vi "IP Units tester V1.vi"() -> ()   [LabVIEW 2015]
uses:
  IP Dev Area/IP results.ctl
  <vilib>/FPGAPlugInAG/Dynamic/niLvFpga_Reset_Dynamic.vi
  <vilib>/FPGAPlugInAG/Dynamic/niLvFpga_Abort_Dynamic.vi
  <vilib>/FPGAPlugInAG/Dynamic/niLvFpga_Run_Dynamic.vi
  <vilib>/Utility/error.llb/Error Cluster From Error Code.vi
  <vilib>/rvi/errors/niLvFpgaAdjustHostInterfaceError.vi
  <vilib>/rvi/interface/common/niFpgaWaitOnOcc.vi
  <vilib>/rvi/interface/nirviMethod/nirviMethod.xnode
  <vilib>/rvi/interface/nirviReadWriteControl/nirviReadWriteControl.xnode
  <vilib>/vision/NI_Vision_Development_Module.lvlib
  <vilib>/rvi/interface/nirviOpenFPGA/nirviOpenFPGA.xnode
  <vilib>/visionFPGA/NI_VDM_FPGA_Basics.lvlib
  <vilib>/visionFPGA/Basics/Configure Image Transfer from Target/IMAQ FPGA Configure Image Transfer from Target U8.vi
  <vilib>/visionFPGA/Basics/Configure Image Transfer to Target/IMAQ FPGA Configure Image Transfer to Target U8.vi
  <vilib>/visionFPGA/Basics/Image Transfer from Target/IMAQ FPGA Image Transfer from Target U8.vi
  <vilib>/rvi/errors/niLvFpgaMergeErrorWithErrorCode.vi
  <vilib>/FPGAPlugInAG/Dynamic/niLvFpga_ConfigureFifo_Dynamic.vi
  <vilib>/FPGAPlugInAG/Dynamic/niLvFpga_StartFifo_Dynamic.vi
  <vilib>/rvi/interface/Simulation/niFpgaSimulationCallBeginRW.vi
  <vilib>/FPGAPlugInAG/Dynamic/niLvFpga_StopFifo_Dynamic.vi
  <vilib>/FPGAPlugInAG/Dynamic/niLvFpga_ReadFifo_Dynamic.vi
  NiFpgaLv.dll
  <vilib>/FPGAPlugInAG/Dynamic/niLvFpga_WriteFifo_Dynamic.vi
  IP Dev Area/FPGA IP Chain V1.vi
  <vilib>/rvi/interface/RandomDataEmulation/nirviRandomDataOpen.vi
  <vilib>/rvi/interface/common/niFpgaCacheSessionInfoDynamic.vi
panel:
  out "SuspPixelsX":u32[](array[numeric])
  out "IP Results":T1
  out "Y Points":i16[](array[numeric])
  out "X Points":i16[](array[numeric])
  out "SuspPixelsIndex":u32[](array[numeric])=[25, 34, 37, 42, 47, 52, 57, 63, 66, 75]
  out "Intensity Graph":u8[][](graph)
  out "ApCounter":u32
  out "Yaccum":u32
  out "Xaccum":u32
  out "counter":u32
  out "error out 7":errorcluster
  out "lo(x)":u16[](array[numeric])
  out "hi(x)":u16[](array[numeric])
  out "error out 6":errorcluster
  out "Results":u32[](array[numeric])
  out "transposed array 2":u8[][](array[numeric])
  out "error out 5":errorcluster
  out "transposed array":u8[][](graph)
  out "error out 4":errorcluster
  out "error out 3":errorcluster
  out "error out 2":errorcluster
  out "error out":errorcluster
  out "Image Out":T2(plugin-control)
  in  "Image Dir Path":path=path "D:/Dropbox (Testview)/Shared Projects/BELKIN Software/Eagle Software/Eagle Code/EyePictures/DebugPics" caption="Image Path"
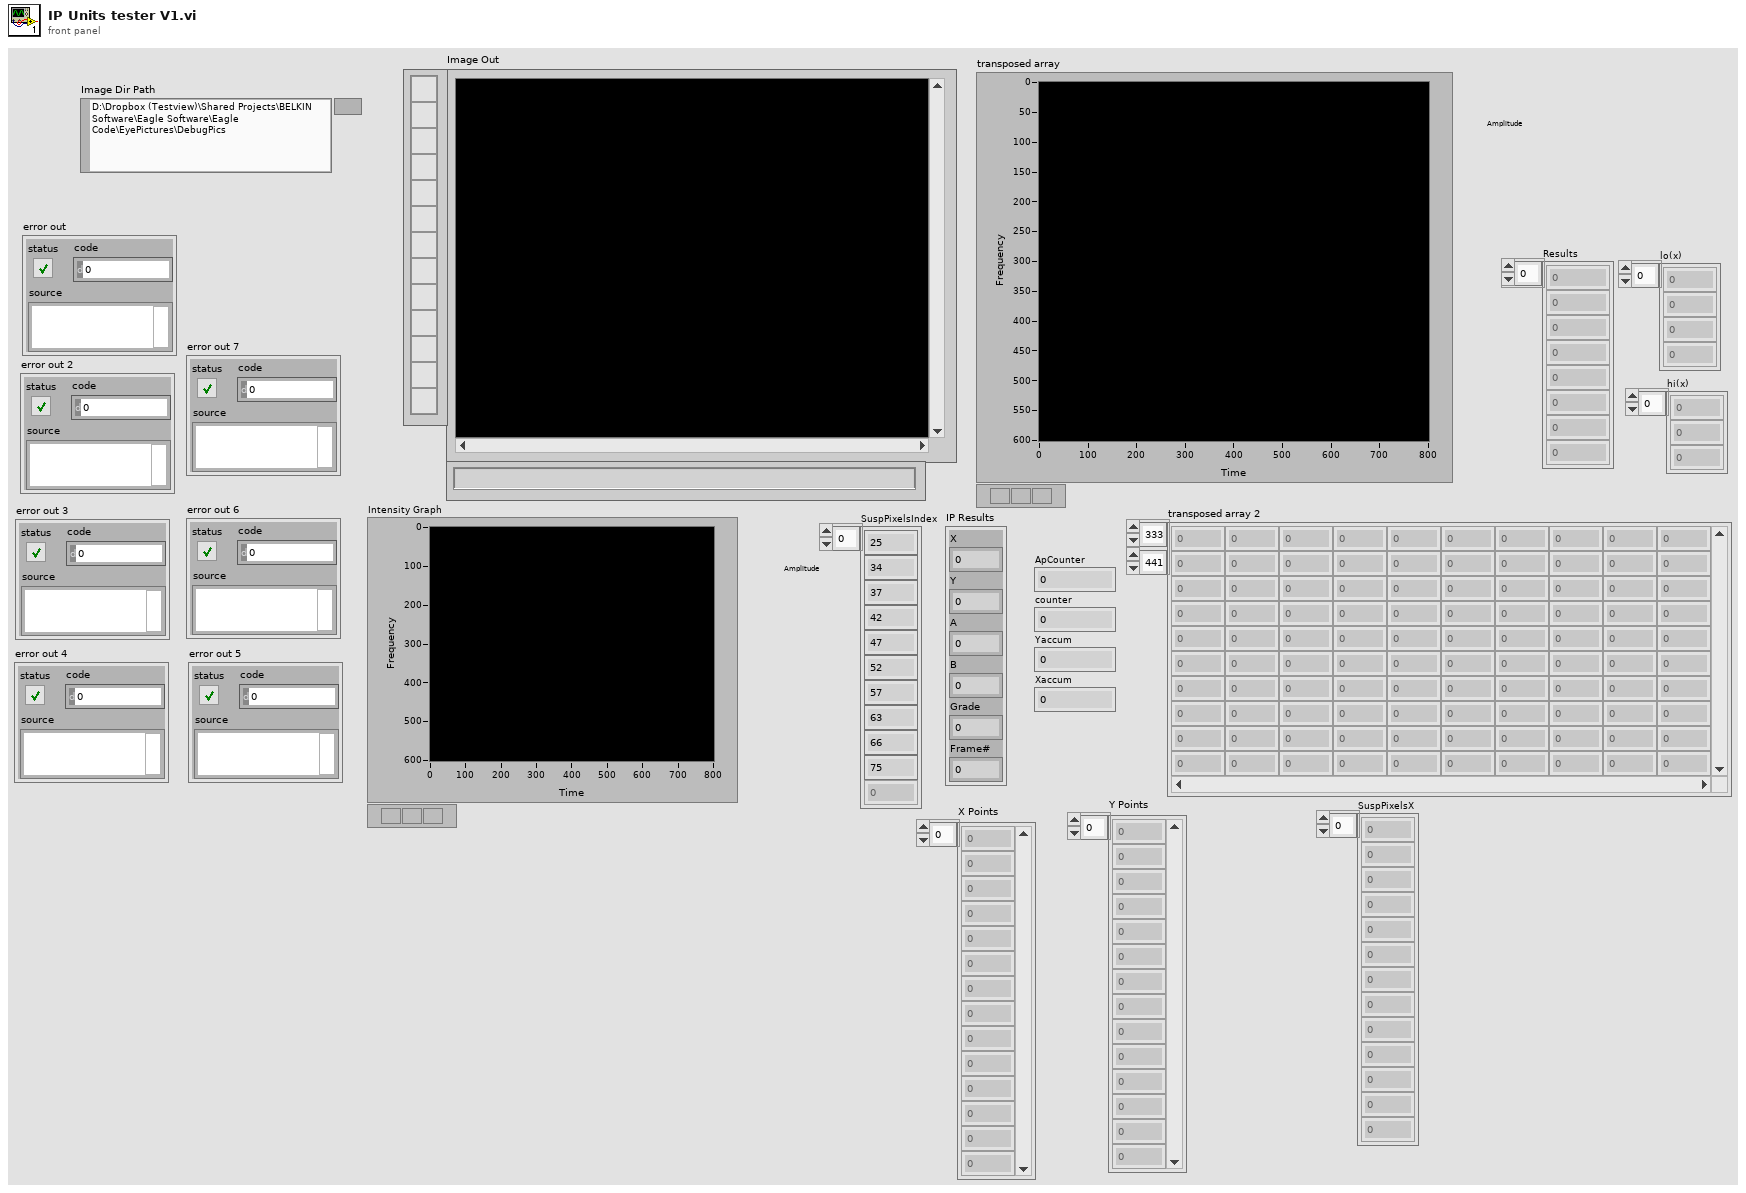
[diagram p1: front panel]
types:
  T1 = typedef "IP results.ctl" = cluster{"X":u16, "Y":u16, "A":dbl, "B":dbl, "Grade":u16, "Frame#":u16}
  T2 = typedef "IMAQ Image.ctl" = refnum<image>
  T3 = typedef "Image Type" = u32
  T4 = cluster{"DMA FIFO Name":string, "Image Size Control Name":string}
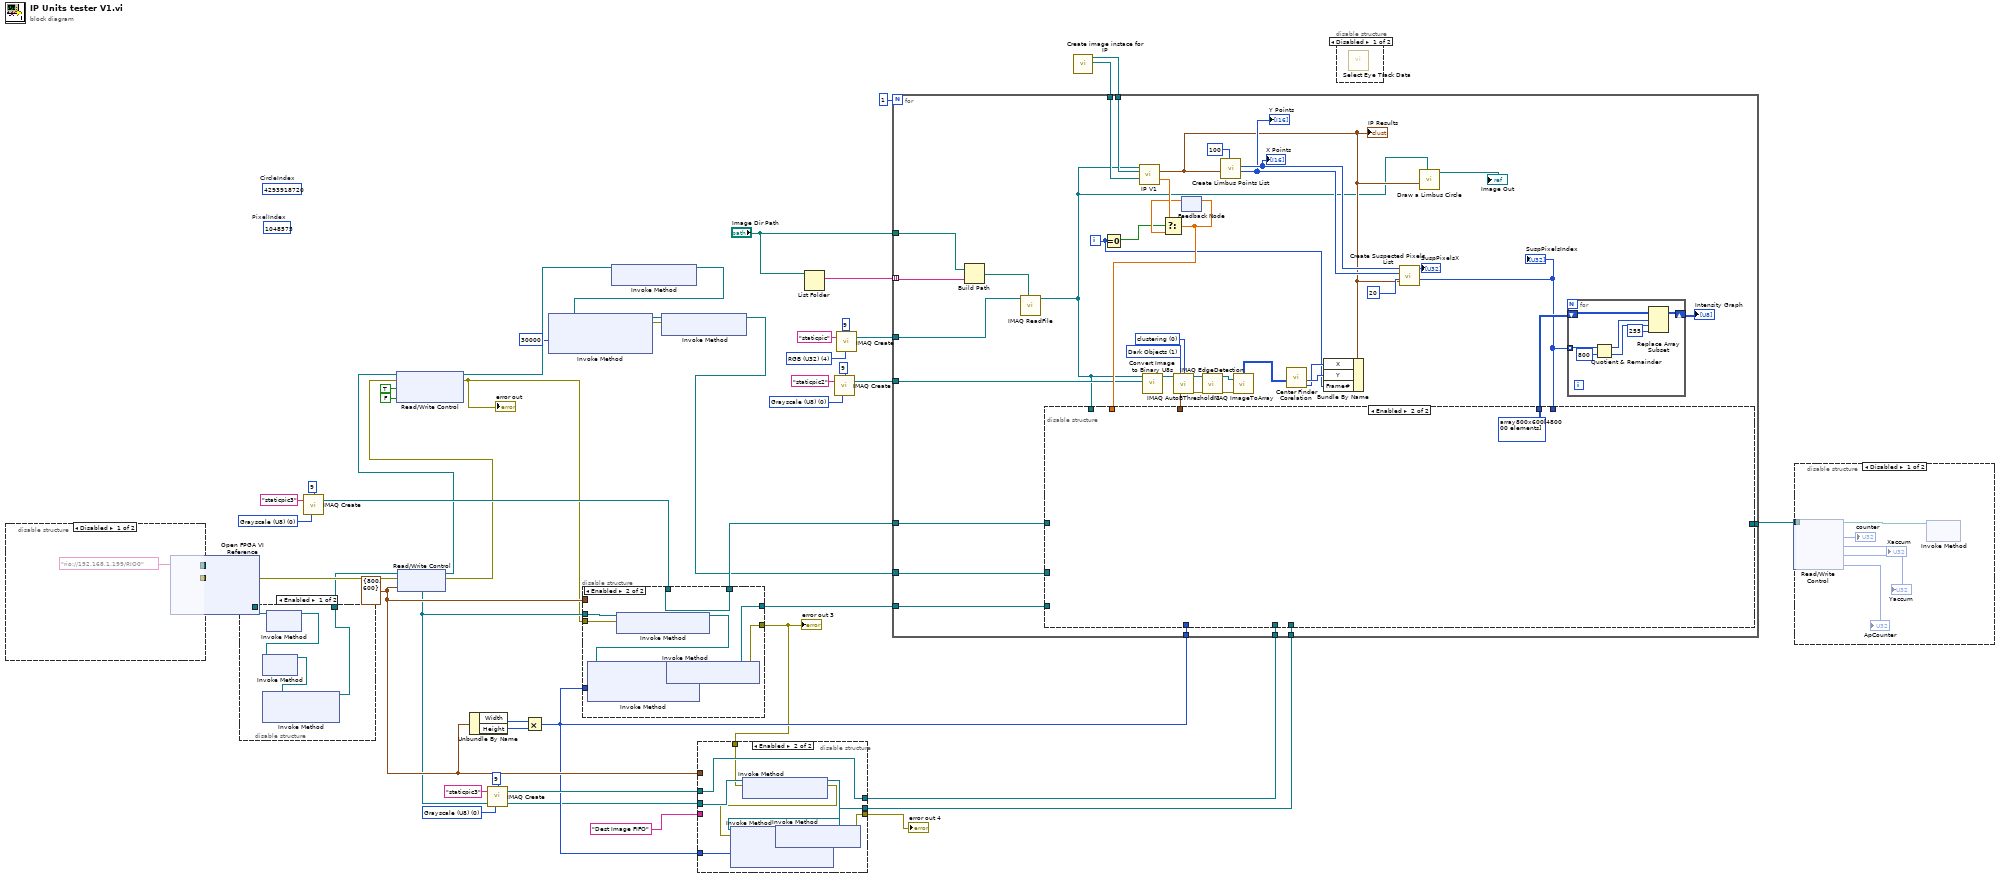
[diagram p0: block diagram]
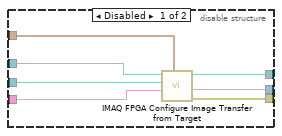
[diagram p6: hidden frame]
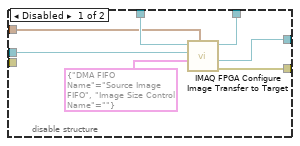
[diagram p7: hidden frame]
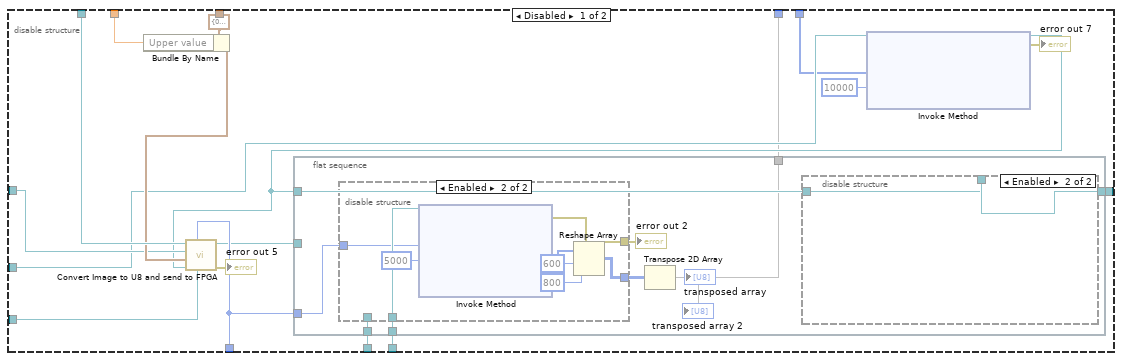
[diagram p8: hidden frame]
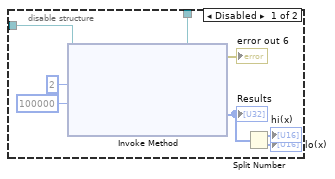
[diagram p9: hidden frame]
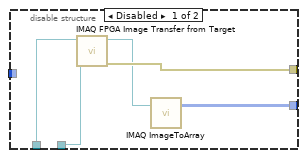
[diagram p10: hidden frame]
diagram:
  (unwired) u32 4293918720  # CircleIndex
  (unwired) u32 1048575  # PixelIndex
  w26 = T3 0 items=["Grayscale (U8)", "Grayscale (I16)", "Grayscale (SGL)", "Complex (CSG)", "RGB (U32)", "HSL (U32)", "RGB (U64)", "Grayscale (U16)"] ("Image Type")
  w19 = cluster{"Width":u32, "Height":u32} {"Width"=800, "Height"=600} ("Image Size")
  w33 = T3 0 items=["Grayscale (U8)", "Grayscale (I16)", "Grayscale (SGL)", "Complex (CSG)", "RGB (U32)", "HSL (U32)", "RGB (U64)", "Grayscale (U16)"] ("Image Type")
  w37 = T3 0 items=["Grayscale (U8)", "Grayscale (I16)", "Grayscale (SGL)", "Complex (CSG)", "RGB (U32)", "HSL (U32)", "RGB (U64)", "Grayscale (U16)"] ("Image Type")
  w44 = T3 4 items=["Grayscale (U8)", "Grayscale (I16)", "Grayscale (SGL)", "Complex (CSG)", "RGB (U32)", "HSL (U32)", "RGB (U64)", "Grayscale (U16)"] ("Image Type")
  n1 = disable-structure shown="Disabled" {
    disable-tunnel: [w49 _] -> w28
    disable-tunnel: [w48 _] -> w2
    frame Disabled {
      n2 = xnode "Open FPGA VI Reference"("resource name"=tag "rio://192.168.1.199/RIO0") -> ("FPGA VI Reference Out"=w48:refnum<k20>, "error out"=w49:errorcluster)  [unwired: 1 in]
    }
    frame Enabled {
    }
  }
  n3 = disable-structure shown="Enabled" {
    disable-tunnel: w2 -> [w54 w55]
    disable-tunnel: [w51 w55] -> w1
    frame Enabled {
      n4 = xnode "Invoke Method"("FPGA VI Reference In"=w54) -> ("FPGA VI Reference Out"=w53:refnum<k20>)  [unwired: 1 in, 1 out]
      n5 = xnode "Invoke Method"("FPGA VI Reference In"=w53) -> ("FPGA VI Reference Out"=w52:refnum<k20>)  [unwired: 1 in, 1 out]
      n6 = xnode "Invoke Method"("FPGA VI Reference In"=w52) -> ("FPGA VI Reference Out"=w51:refnum<k20>)  [unwired: 2 in, 1 out]
    }
    frame Disabled {
    }
  }
  n7 = call "IMAQ Create"("Border Size"=9, "Image Name"="staticpic3", "Image Type"=w33) -> ("New Image"=w30:T2)  [unwired: 1 in, 2 out]
  n8 = xnode "Read/Write Control"("FPGA VI Reference In"=w1, "error in"=w28, "Image Size"=w19) -> ("FPGA VI Reference Out"=w15:refnum<k20>, "error out"=w13:errorcluster)
  n9 = xnode "Read/Write Control"("FPGA VI Reference In"=w15, "error in"=w13, "ResetAPCounter"=TRUE, "ResetAPCounter"=FALSE) -> ("FPGA VI Reference Out"=w6:refnum<k20>, "error out"=w10:errorcluster)
  "error out" <- w10
  n10 = Unbundle By Name(w19) -> ("Width"=w18:u32, "Height"=w17:u32)
  n11 = call "IMAQ Create"("Border Size"=9, "Image Name"="staticpic3", "Image Type"=w26) -> ("New Image"=w24:T2)  [unwired: 1 in, 2 out]
  n12 = Multiply(x=w18, y=w17) -> (x*y=w16:u32)
  n13 = disable-structure shown="Enabled" {
    disable-tunnel: [w62 w68] -> w31
    disable-tunnel: w30 -> [w61 w71]
    disable-tunnel: [w60 w71] -> w29
    disable-tunnel: [w58 w66] -> w12
    disable-tunnel: w15 -> [w57 w65]
    disable-tunnel: w19 -> [w56 _]
    disable-tunnel: w16 -> [_ w69]
    disable-tunnel: w10 -> [_ w63]
    frame Disabled {
      n14 = call-poly <vilib>:"IMAQ FPGA Configure Image Transfer to Target.vi"("Image Size"=w56, "Resource Names"=T4 {"DMA FIFO Name"="Source Image FIFO", "Image Size Control Name"=""}, "FPGA VI Reference In"=w57, "Image"=w61) -> ("error out"=w58:errorcluster, "DMA FIFO Reference Out"=w62:refnum<k20>, "Image Out"=w60:T2)  [unwired: 4 in, 1 out]
    }
    frame Enabled {
      n15 = xnode "Invoke Method"("FPGA VI Reference In"=w65, "error in"=w63) -> ("FPGA VI Reference Out"=w64:refnum<k20>)  [unwired: 1 out]
      n16 = xnode "Invoke Method"("FPGA VI Reference In"=w64, "Requested Depth"=w69) -> ("FPGA VI Reference Out"=w70:refnum<k20>, "error out"=w67:errorcluster)  [unwired: 1 in, 1 out]
      n17 = xnode "Invoke Method"("FPGA VI Reference In"=w70, "error in"=w67) -> ("FPGA VI Reference Out"=w68:refnum<k20>, "error out"=w66:errorcluster)
    }
  }
  "error out 3" <- w12
  n18 = xnode "Invoke Method"("FPGA VI Reference In"=w6) -> ("FPGA VI Reference Out"=w7:refnum<k20>)  [unwired: 1 in, 1 out]
  n19 = xnode "Invoke Method"("FPGA VI Reference In"=w7, "Requested Depth"=u32 30000) -> ("FPGA VI Reference Out"=w8:refnum<k20>, "error out"=w9:errorcluster)  [unwired: 1 in, 1 out]
  n20 = xnode "Invoke Method"("FPGA VI Reference In"=w8, "error in"=w9) -> ("FPGA VI Reference Out"=w5:refnum<k20>)  [unwired: 1 out]
  n21 = disable-structure shown="Enabled" {
    disable-tunnel: w24 -> [w78 w88]
    disable-tunnel: w15 -> [w77 w83]
    disable-tunnel: [w76 w88] -> w23
    disable-tunnel: [w75 w84] -> w22
    disable-tunnel: [w74 w81] -> w21
    disable-tunnel: "Dest Image FIFO" ("DMA FIFO Name") -> [w73 _]
    disable-tunnel: w19 -> [w72 _]
    disable-tunnel: w16 -> [_ w85]
    disable-tunnel: w12 -> [_ w79]
    frame Disabled {
      n22 = call-poly <vilib>:"IMAQ FPGA Configure Image Transfer from Target.vi"("Image Size"=w72, "DMA FIFO Name"=w73, "FPGA VI Reference In"=w77, "Image"=w78) -> ("error out"=w74:errorcluster, "DMA FIFO Reference Out"=w75:refnum<k20>, "Image Out"=w76:T2)  [unwired: 5 in]
    }
    frame Enabled {
      n23 = xnode "Invoke Method"("FPGA VI Reference In"=w83, "error in"=w79) -> ("FPGA VI Reference Out"=w82:refnum<k20>, "error out"=w80:errorcluster)
      n24 = xnode "Invoke Method"("FPGA VI Reference In"=w82, "error in"=w80, "Requested Depth"=w85) -> ("FPGA VI Reference Out"=w86:refnum<k20>, "error out"=w87:errorcluster)  [unwired: 1 out]
      n25 = xnode "Invoke Method"("FPGA VI Reference In"=w86, "error in"=w87) -> ("FPGA VI Reference Out"=w84:refnum<k20>, "error out"=w81:errorcluster)
    }
  }
  "error out 4" <- w21
  n26 = List Folder(path="Image Dir Path") -> (filenames=w47:string[])  [unwired: 3 in, 3 out]
  n27 = call "IMAQ Create"("Border Size"=9, "Image Name"="staticpic2", "Image Type"=w37) -> ("New Image"=w39:T2)  [unwired: 1 in, 2 out]
  n28 = call "IMAQ Create"("Border Size"=9, "Image Name"="staticpic", "Image Type"=w44) -> ("New Image"=w42:T2)  [unwired: 1 in, 2 out]
  n29 = call "Create image instace for IP.vi"() -> ("Zoom"=w41:T2, "algo2"=w40:T2)  [unwired: 9 in, 1 out]
  n30 = for {
    N: 1 -> [_]
    tunnel: w47 -> [w121] mode=indexing
    tunnel: "Image Dir Path" -> [w120]
    tunnel: w42 -> [w119]
    tunnel: w41 -> [w118]
    tunnel: w40 -> [w117]
    tunnel: w39 -> [w107]
    tunnel: w5 -> [w98]
    tunnel: w29 -> [w105]
    tunnel: [w104] -> w3
    tunnel: w31 -> [w99]
    tunnel: w23 -> [w103]
    tunnel: w22 -> [w102]
    tunnel: w16 -> [w101]
    i -> [w109]
    w126 = 0 items=["clustering", "entropy", "metric", "moments", "inter-class variance"] ("Method (clustering)")
    w125 = u32 1 items=["Bright Objects", "Dark Objects"] ("Look For (Bright Objects)")
    n31 = Build Path(base path=w120, name or relative path=w121) -> (appended path=w122:path)
    n32 = call "IMAQ ReadFile"("File Path"=w122, "Image"=w119) -> ("Image Out"=w90:T2)  [unwired: 3 in, 6 out]
    n33 = Equal To 0?(x=w109) -> (x = 0?=w110:bool)
    n34 = call "IP V1.vi"("Image In"=w90, "Image Dst"=w117, "Zoom Image"=w118) -> ("IP Results"=w91:T1, "ThreshOut"=w115:sgl)  [unwired: 9 in, 2 out]
    "IP Results" <- w91
    n35 = call "Convert Image to Binary U8s.vi"("Image Dst"=w107, "ImageIn"=w90) -> ("Image Out"=w108:T2)  [unwired: 8 in, 1 out]
    n36 = feedback #1() -> (w113:sgl)  [unwired: 1 in]
    n37 = Select(t=w115, s=w110, f=w113) -> (s? t:f=w114:sgl)
    n38 = feedback-in #1(w114) -> ()
    n39 = call "Create Limbus Points List.vi"("NoOfPoints"=u16 100, "IP Results"=w91) -> ("Y Points"=w92:i16[], "X Points"=w93:i16[])  [unwired: 8 in]
    "X Points" <- w93
    "Y Points" <- w92
    n40 = call "Create Suspected Pixels List.vi"("IP Results"=w91, "tolerance"=20, "Y Points"=w92, "X Points"=w93) -> ("SuspPixelsIndex"=w95:u32[], "SuspPixelsX"=→"SuspPixelsX":u32[])  [unwired: 5 in, 1 out]
    "SuspPixelsIndex" <- w95
    n41 = disable-structure shown="Enabled" {
      disable-tunnel: w114 -> [w147 _]
      disable-tunnel: w90 -> [w145 _]
      disable-tunnel: [w144 _] -> w106
      disable-tunnel: w105 -> [w143 _]
      disable-tunnel: [w142 _] -> w104
      disable-tunnel: w103 -> [w141 _]
      disable-tunnel: w102 -> [w140 _]
      disable-tunnel: w101 -> [w139 _]
      disable-tunnel: w99 -> [w137 _]
      disable-tunnel: w98 -> [w136 _]
      disable-tunnel: [w133 u8[][] array800x600[480000 elements]] -> w96
      disable-tunnel: w95 -> [w132 _]
      frame Disabled {
        n42 = Bundle By Name(cluster=cluster{"Lower value":sgl, "Upper value":sgl} {"Lower value"=0.0, "Upper value"=255.0} ("Threshold Limits"), "Upper value"=w147) -> (w144:cluster{"Lower value":sgl, "Upper value":sgl})
        n43 = flat-sequence {
          tunnel: w134 -> [w151]
          tunnel: w131 -> [_]
          tunnel: [w149] -> w142
          tunnel: w141 -> [w155]
          tunnel: w140 -> [w154]
          tunnel: w139 -> [w152]
          tunnel: [w148] -> w133
          frame #0 {
            n44 = disable-structure shown="Enabled" {
              disable-tunnel: w155 -> [w169 _]
              disable-tunnel: w154 -> [w168 w177]
              disable-tunnel: [w167 w172] -> w150
              disable-tunnel: [w165 w173] -> w153
              disable-tunnel: w152 -> [_ w170]
              frame Disabled {
                n45 = call-poly <vilib>:"IMAQ FPGA Image Transfer from Target.vi"("DMA FIFO Reference In"=w168, "Image"=w169) -> ("error out"=w167:errorcluster, "Image Out"=w166:T2)  [unwired: 7 in, 1 out]
                n46 = call "IMAQ ImageToArray"("Image"=w166) -> ("Image Pixels (U8)"=w165:u8[][])  [unwired: 3 in, 4 out]
              }
              frame Enabled {
                n47 = xnode "Invoke Method"("FPGA VI Reference In"=w177, "Number of Elements"=w170, "Timeout (ms)"=5000) -> ("error out"=w172:errorcluster, "Data"=w176:u8[])  [unwired: 1 in, 2 out]
                n48 = Reshape Array(w176, 600 ("dimension size"), 800 ("dimension size")) -> (w173:u8[][])
              }
            }
            "error out 2" <- w150
            n49 = Transpose 2D Array(2D array=w153) -> (transposed array=w148:u8[][])
            "transposed array" <- w148
            "transposed array 2" <- w148
            n50 = disable-structure shown="Enabled" {
              disable-tunnel: w151 -> [w163 w164]
              disable-tunnel: [w160 w164] -> w149
              frame Disabled {
                n51 = xnode "Invoke Method"("FPGA VI Reference In"=w163, "Number of Elements"=u32 2, "Timeout (ms)"=100000) -> ("FPGA VI Reference Out"=w160:refnum<k20>, "error out"=→"error out 6":errorcluster, "Data"=w158:u32[])  [unwired: 1 in, 1 out]
                "Results" <- w158
                n52 = Split Number(x=w158) -> (hi(x)=→"hi(x)":u16[], lo(x)=→"lo(x)":u16[])
              }
              frame Enabled {
              }
            }
          }
        }
        n53 = xnode "Invoke Method"("FPGA VI Reference In"=w136, "Data"=w132, "Timeout (ms)"=10000) -> ("FPGA VI Reference Out"=w134:refnum<k20>, "error out"=→"error out 7":errorcluster)  [unwired: 1 in, 1 out]
        n54 = call "Convert Image to U8 and send to FPGA.vi"(6:"FPGA VI Reference Out 2"=w137, "Maximum Pixels per Write"=w139, 8:"FPGA VI Reference Out 2"=w134, "Range"=w144, "Image Dst"=w143, "ImageIn"=w145) -> ("error out"=→"error out 5":errorcluster, "Image Out"=w131:T2)  [unwired: 3 in, 1 out]
      }
      frame Enabled {
      }
    }
    n55 = call "IMAQ AutoBThreshold 2"("Image Src"=w108, "Look For (Bright Objects)"=w125, "Method (clustering)"=w126, "Threshold Limits"=w106) -> ("Image Dst Out"=w124:T2, "error out"=w123:errorcluster)  [unwired: 9 in, 1 out]
    n56 = call "IMAQ EdgeDetection"("error in (no error)"=w123, "Image Src"=w124) -> ("error out"=w127:errorcluster, "Image Dst Out"=w129:T2)  [unwired: 8 in]
    n57 = call "IMAQ ImageToArray"("error in (no error)"=w127, "Image"=w129) -> ("Image Pixels (U8)"=w128:u8[][])  [unwired: 2 in, 4 out]
    n58 = call "Center Finder Corelation.vi"("Picture"=w128) -> ("X"=w111:u32, "Y"=w112:u32)  [unwired: 8 in, 1 out]
    n59 = Bundle By Name(cluster=w91, "X"=w111, "Y"=w112, "Frame#"=w109) -> ()  [unwired: 1 out]
    n60 = call "Draw a Limbus Circle.vi"("Img In"=w90, "IP Results"=w91) -> ("Img Out"=→"Image Out":T2)  [unwired: 8 in, 1 out]
    n61 = for {
      tunnel: w95 -> [w185] mode=indexing
      shift-right: [w182] -> w97
      shift-left: w96 -> [w183]
      n62 = Quotient & Remainder(x=w185, y=u32 800) -> (x-y*floor(x/y)=w179:u32, floor(x/y)=w180:u32)
      n63 = Replace Array Subset(array=w183, new element=u8 255 ("new element/subarray"), index (row)=w179, index (col)=w180) -> (w182:u8[][])
    }
    "Intensity Graph" <- w97
  }
  n64 = disable-structure shown="Disabled" {
    frame Disabled {
      n65 = call "Select Eye Track Data.vi"() -> ()  [unwired: 8 in, 4 out]
    }
    frame Enabled {
    }
  }
  n66 = disable-structure shown="Disabled" {
    disable-tunnel: w3 -> [w191 _]
    frame Disabled {
      n67 = xnode "Read/Write Control"("FPGA VI Reference In"=w191) -> ("FPGA VI Reference Out"=w190:refnum<k20>, "counter"=→"counter":u32, "Xaccum"=→"Xaccum":u32, "Yaccum"=→"Yaccum":u32, "ApCounter"=→"ApCounter":u32)  [unwired: 1 in, 1 out]
      n68 = xnode "Invoke Method"("FPGA VI Reference In"=w190) -> ()  [unwired: 1 in, 2 out]
    }
    frame Enabled {
    }
  }
